vi "Get SLSC Switch Slot Number.vi"(8 "error in":errorcluster, 11 "slsc switch custom device in":T1 format="%.0x") -> (0 "error out":errorcluster, 2 "slot number":i32, 3 "slsc switch custom device out":T1 format="%.0x")   [LabVIEW 2017, in "NI-SWITCH Scripting.lvlib"]
uses:
  NI-SWITCH Scripting.lvlib
  SLSC Scripting Constants.vi
  <vilib>/NI VeriStand/Custom Device API/Custom Device API.lvlib
  <vilib>/NI Veristand/Custom Device API/Get Item Property (I32).vi
  <vilib>/NI Veristand/Custom Device API/Custom Device Item Ref.ctl
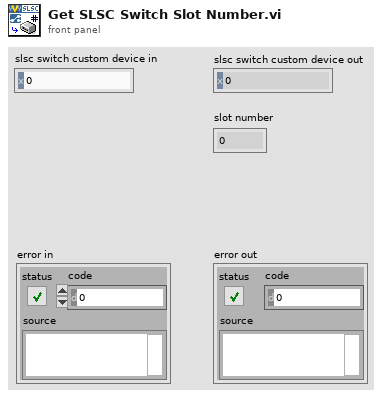
[diagram p1: front panel]
types:
  T1 = typedef "Custom Device API.lvlib/Custom Device Item Ref.ctl" = u64
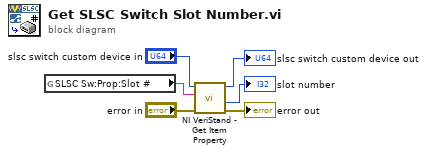
[diagram p0: block diagram]
diagram:
  n1 = global read "SLSC Scripting Constants.vi" "SLSC Sw:Prop:Slot #"() -> (w3:string)
  n2 = call-poly <vilib>:"NI VeriStand - Get Item Property.vi"("error in (no error)"="error in", "Property Name"=w3, "Item Ref in"="slsc switch custom device in") -> ("error out"=→"error out":errorcluster, "Value"=→"slot number":i32, "Item Ref out"=→"slsc switch custom device out":T1)  [unwired: 5 in, 1 out]
